vi "Create Gate.vi"(0 "Ramp (ms)":dbl, 5 "Duration (ms)":dbl, 7 "Sampling Rate (Hz)":dbl, 9 "Npts":i32, 11 "error in (no error)":errorcluster) -> (8 "Gate":dbl[](array[numeric]), 15 "error out":errorcluster)   [LabVIEW 2020]
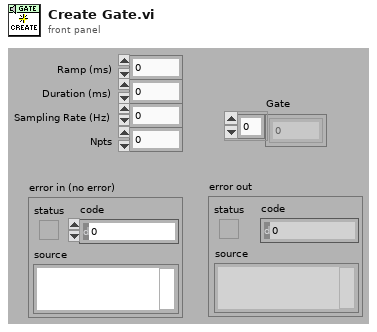
[diagram p1: front panel]
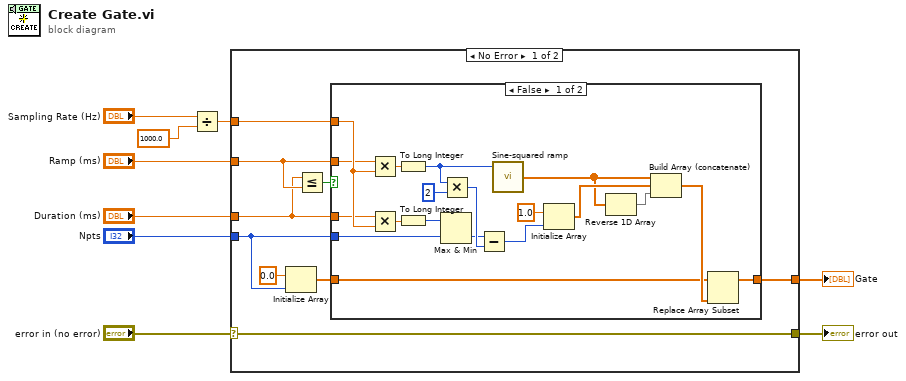
[diagram p0: block diagram]
diagram:
  n1 = Divide(x="Sampling Rate (Hz)", y=1000.0) -> (x/y=w4:dbl)
  n2 = case shown="No Error" "error in (no error)" {
    selector: "error in (no error)" -> [w14 w39]
    tunnel: [w18 _] -> w8
    tunnel: [w14 w39] -> w7
    tunnel: "Ramp (ms)" -> [w17 _]
    tunnel: w4 -> [w16 _]
    tunnel: "Duration (ms)" -> [w15 _]
    tunnel: "Npts" -> [w10 _]
    frame No Error {
      n3 = Initialize Array(0.0 ("element"), w10) -> (w11:dbl[])
      n4 = Less Or Equal?(x=w15, y=w17) -> (x <= y?=w13:bool)
      n5 = case shown="False" w13 {
        tunnel: w16 -> [w28 _]
        tunnel: [w27 w38] -> w18
        tunnel: w17 -> [w26 _]
        tunnel: w15 -> [w25 _]
        tunnel: w11 -> [w22 w38]
        tunnel: w10 -> [w20 _]
        frame False {
          n6 = Multiply(x=w26, y=w28) -> (x*y=w37:dbl)
          n7 = Multiply(x=w25, y=w28) -> (x*y=w34:dbl)
          n8 = To Long Integer(number=w37) -> (32bit integer=w36:i32)
          n9 = To Long Integer(number=w34) -> (32bit integer=w21:i32)
          n10 = Max & Min(x=w21, y=w20) -> (min(x,y)=w19:i32)  [unwired: 1 out]
          n11 = Multiply(x=w36, y=2) -> (x*y=w33:i32)
          n12 = Subtract(x=w19, y=w33) -> (x-y=w32:i32)
          n13 = call "Sine-squared ramp.vi"("samples"=w36) -> ("sine^2 Ramp"=w24:dbl[])  [unwired: 3 in, 1 out]
          n14 = Initialize Array(1.0 ("element"), w32) -> (w30:dbl[])
          n15 = Reverse 1D Array(array=w24) -> (reversed array=w29:dbl[])
          n16 = Build Array (concatenate)(w24, w30, w29) -> (w23:dbl[])
          n17 = Replace Array Subset(array=w22, new element=w23) -> (w27:dbl[])  [unwired: 1 in]
        }
        frame True {
        }
      }
    }
    frame Error {
    }
  }
  "error out" <- w7
  "Gate" <- w8
